vi "DOCK_MAIN_check_for_error.vi"(8 "MAIN_loop_state_in":T1, 11 "error_in":errorcluster) -> (0 "MAIN_loop_state_out":T1, 3 "error_out":errorcluster)   [LabVIEW 2019]
uses:
  DOCK_MAIN_sequence_state.ctl
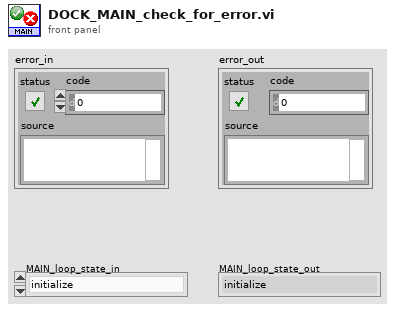
[diagram p1: front panel]
types:
  T1 = typedef "DOCK_MAIN_sequence_state.ctl" = enum16{"initialize", "get_next_state", "USER_login", "USER_logout", "read_reference_list", "read_batch_size_list", "change_reference", "start_batch", "reload_batch", "finish_batch?", "finish_batch", "preread_gear_data_check", "read_gear_data", "refresh_gear_data", "save_gear_to_batch", "clear_gear_data", "print_label", "report_get", "error", "stop"}
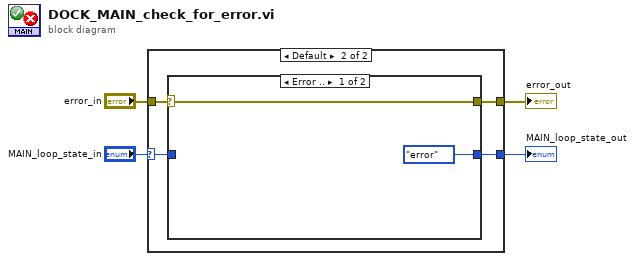
[diagram p0: block diagram]
diagram:
  n1 = case shown="Default" "MAIN_loop_state_in" {
    selector: "MAIN_loop_state_in" -> [w6 w8]
    tunnel: [w5 w10] -> w4
    tunnel: [w6 w9] -> w3
    tunnel: "error_in" -> [w5 w7]
    frame "stop" {
    }
    frame Default {
      n2 = case shown="Error .." w7 {
        selector: w7 -> [w12 w13]
        tunnel: [DOCK_MAIN_sequence_state."error" ("MAIN_loop_state_in") w14] -> w9
        tunnel: w8 -> [_ w14]
        tunnel: [w12 w13] -> w10
        frame Error {
        }
        frame No Error {
        }
      }
    }
  }
  "error_out" <- w4
  "MAIN_loop_state_out" <- w3
